vi "Image Processing with Vision Assistant (FPGA)test.vi"() -> ()   [LabVIEW 2016]
uses:
  <vilib>/visionFPGA/Controls/IMAQ FPGA Image Size.ctl
  <vilib>/rvi/Emulation/niFpgaSctlEmulationGetInTimedLoop.vi
  <vilib>/rvi/Emulation/niFpgaProcessEmulError.vi
  <vilib>/rvi/Emulation/niFpgaGetClockAttributes.vi
  <vilib>/rvi/Emulation/niFpgaEmulationReportErrorSimple.vi
  <vilib>/visionFPGA/Basics/FIFO to Pixel Bus/IMAQ FPGA FIFO to Pixel Bus RGB32x1.vi
  <vilib>/rvi/DataTransferAndStorage/Container/Common/niFpgaContainerGetUniqueNameForEmu.vi
  <vilib>/rvi/DataTransferAndStorage/Container/Common/niFpgaContainerSetEmuInfo.vi
  <vilib>/rvi/eio/common/nirviEmuReportErrorAndStop.vi
  <vilib>/rvi/interface/RandomDataEmulation/niFpgaRandomDataHandleErrors.vi
  <vilib>/rvi/Emulation/niFpgaCriticalErrorInLSC.vi
  <vilib>/rvi/LocalResourceManager/LocalResourceManager.xnode
  <vilib>/rvi/DataTransferAndStorage/Container/XNode/niFpgaContainer.xnode
  <vilib>/rvi/interface/RandomDataEmulation/nirviRandomDataFpgaReadWriteTemplate.vi
  <vilib>/visionFPGA/NI_VDM_FPGA_Basics.lvlib
panel:
  out "Output Valid":bool
  out "Ready For Output":bool=TRUE
  out "StartOfImage":bool=TRUE
  in  "Image Size":T1={"Width"=640, "Height"=480}
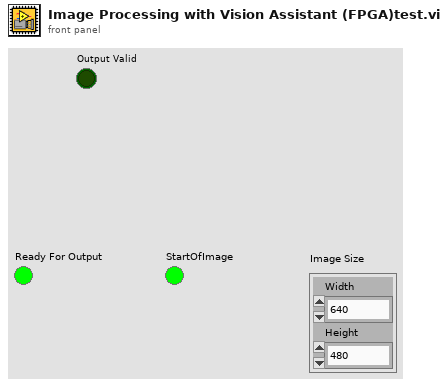
[diagram p1: front panel]
types:
  T1 = typedef "IMAQ FPGA Image Size.ctl" = cluster{"Width":u32, "Height":u32}
  T2 = typedef "IMAQ FPGA Pixel Bus RGB32x1.ctl" = cluster{"Pixel Data":cluster{"A":u8, "R/H":u8, "G/S":u8, "B/L":u8}, "DV":bool, "EOL":bool, "EOI":bool, "Data Type":enum16{"RGB32 x 1"}}
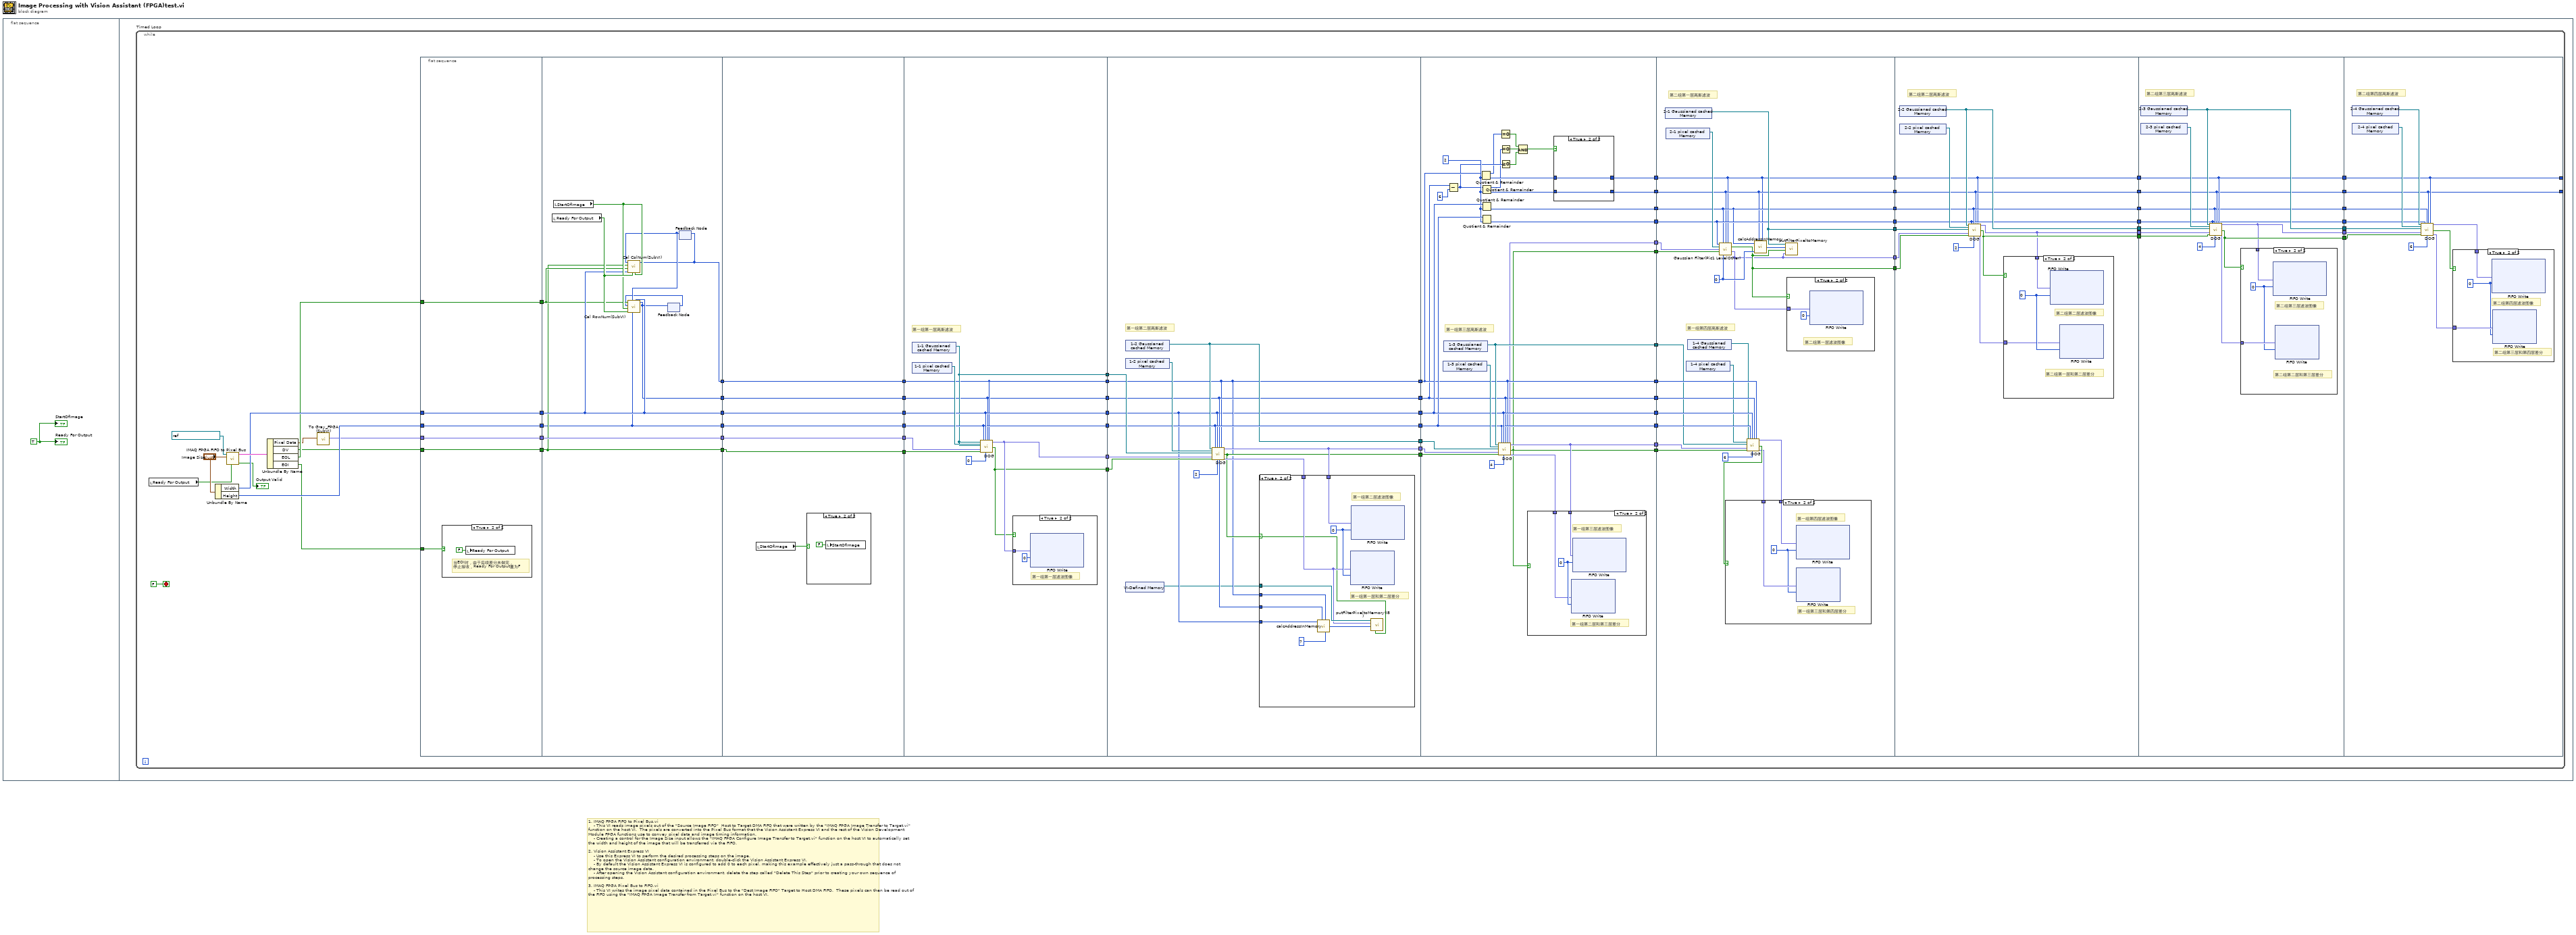
[diagram p0: block diagram]
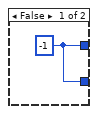
[diagram p6: hidden frame]
diagram:
  # "1. IMAQ FPGA FIFO to Pixel Bus.vi\n    - This VI reads image pixels out of the \"Source Image FIFO\"  Host to Target DMA FIFO that were written by the \"IMAQ FPGA Image Transfer to Target.vi\" function on the host VI.  The pixels are converted into the Pixel Bus format that the Vision Assistant Express VI and the rest of the Vision Development Module FPGA functions use to convey pixel data and image timing information.\n    - Creating a control for the Image Size input allows the \"IMAQ FPGA Configure Image Transfer to Target.vi\" function on the host VI to automatically set the width and height of the image that will be transferred via the FIFO.\n\n2. Vision Assistant Express VI\n    - Use this Express VI to perform the desired processing steps on the image.\n    - To open the Vision Assistant configuration environment, double-click the Vision Assistant Express VI.\n    - By default the Vision Assistant Express VI is configured to add 0 to each pixel, making this example effectively just a pass-through that does not change the source image data.\n    - After opening the Vision Assistant configuration environment, delete the step called \"Delete This Step\" prior to creating your own sequence of processing steps.\n\n3. IMAQ FPGA Pixel Bus to FIFO.vi\n    - This VI writes the image pixel data contained in the Pixel Bus to the \"Dest Image FIFO\" Target to Host DMA FIFO.  These pixels can then be read out of the FIFO using the \"IMAQ FPGA Image Transfer from Target.vi\" function on the host VI."
  n1 = flat-sequence {
    frame #0 {
      w1 = TRUE ("Ready For Output")
      "StartOfImage" <- w1
      "Ready For Output" <- w1
    }
    frame #1 {
      n2 = while "Timed Loop" {
        stop <- FALSE stop-if-true
        n3 = local read "Ready For Output"() -> (w12:bool)
        n4 = Unbundle By Name("Image Size") -> ("Width"=w68:u32, "Height"=w76:u32)
        n5 = call-poly <vilib>:"IMAQ FPGA FIFO to Pixel Bus.vi"("Ready For Output"=w12, "Image Size"="Image Size", "Source Image FIFO"=refnum<k21> "32it Source FIFO") -> ("Output Valid"=→"Output Valid":bool, "Pixel Bus Out"=w78:T2)  [unwired: 6 in, 1 out]
        n6 = Unbundle By Name(w78) -> ("Pixel Data"=w3:cluster{"A":u8, "R/H":u8, "G/S":u8, "B/L":u8}, "DV"=w2:bool, "EOL"=w13:bool, "EOI"=w75:bool)
        n7 = call "To Gray_FPGA (SubVI).vi"("Pixel Data"=w3) -> ("Data Out"=w4:fxp<+,8,8>)  [unwired: 10 in]
        n8 = flat-sequence {
          tunnel: w13 -> [w81]
          tunnel: w75 -> [w80]
          tunnel: w2 -> [w82]
          tunnel: w76 -> [w83]
          tunnel: w68 -> [w84]
          tunnel: w4 -> [w85]
          tunnel: [w85] -> w11
          tunnel: [w84] -> w10
          tunnel: [w83] -> w9
          tunnel: [w82] -> w8
          tunnel: [w81] -> w7
          tunnel: [w89] -> w19
          tunnel: [w87] -> w18
          tunnel: [w97] -> w17
          tunnel: [w94] -> w16
          tunnel: [w91] -> w15
          tunnel: [w92] -> w14
          tunnel: w11 -> [w97]
          tunnel: w10 -> [w94]
          tunnel: w9 -> [w91]
          tunnel: w8 -> [w92]
          tunnel: w7 -> [w93]
          tunnel: [w98] -> w74
          tunnel: [w104] -> w73
          tunnel: [w102] -> w72
          tunnel: [w103] -> w71
          tunnel: [w100] -> w70
          tunnel: [w99] -> w69
          tunnel: w19 -> [w99]
          tunnel: w18 -> [w100]
          tunnel: w17 -> [w104]
          tunnel: w16 -> [w103]
          tunnel: w15 -> [w102]
          tunnel: w14 -> [w98]
          tunnel: w74 -> [w115]
          tunnel: w73 -> [w116]
          tunnel: w72 -> [w111]
          tunnel: w71 -> [w112]
          tunnel: w70 -> [w107]
          tunnel: w69 -> [w106]
          tunnel: [w107] -> w67
          tunnel: [w106] -> w66
          tunnel: [w112] -> w65
          tunnel: [w111] -> w64
          tunnel: [w114] -> w63
          tunnel: [w108] -> w62
          tunnel: [w109] -> w59
          tunnel: w67 -> [w121]
          tunnel: w66 -> [w126]
          tunnel: w65 -> [w120]
          tunnel: w64 -> [w128]
          tunnel: w63 -> [w130]
          tunnel: w62 -> [w129]
          tunnel: [w123] -> w61
          tunnel: [w125] -> w60
          tunnel: w59 -> [w131]
          tunnel: [w121] -> w58
          tunnel: [w126] -> w57
          tunnel: [w120] -> w56
          tunnel: [w128] -> w55
          tunnel: [w127] -> w47
          tunnel: w61 -> [w171]
          tunnel: w60 -> [w170]
          tunnel: w58 -> [w159]
          tunnel: w57 -> [w158]
          tunnel: w56 -> [w164]
          tunnel: w55 -> [w162]
          tunnel: [w146] -> w54
          tunnel: [w144] -> w53
          tunnel: [w159] -> w52
          tunnel: [w158] -> w51
          tunnel: [w164] -> w50
          tunnel: [w162] -> w49
          tunnel: [w168] -> w48
          tunnel: w47 -> [w167]
          tunnel: [w163] -> w46
          tunnel: [w160] -> w45
          tunnel: [w152] -> w44
          tunnel: [w153] -> w43
          tunnel: [w146] -> w42
          tunnel: [w144] -> w41
          tunnel: w54 -> [w202]
          tunnel: w53 -> [w201]
          tunnel: w52 -> [w200]
          tunnel: w51 -> [w199]
          tunnel: w50 -> [w198]
          tunnel: w49 -> [w197]
          tunnel: w48 -> [w194]
          tunnel: w46 -> [w185]
          tunnel: w45 -> [w186]
          tunnel: w44 -> [w184]
          tunnel: w43 -> [w183]
          tunnel: w42 -> [w188]
          tunnel: w41 -> [w189]
          tunnel: [w191] -> w40
          tunnel: [w180] -> w39
          tunnel: [w181] -> w38
          tunnel: [w186] -> w37
          tunnel: [w185] -> w36
          tunnel: [w184] -> w35
          tunnel: [w183] -> w34
          tunnel: w40 -> [w218]
          tunnel: w39 -> [w217]
          tunnel: w38 -> [w216]
          tunnel: w37 -> [w213]
          tunnel: w36 -> [w214]
          tunnel: w35 -> [w212]
          tunnel: w34 -> [w211]
          tunnel: [w215] -> w33
          tunnel: [w211] -> w32
          tunnel: [w212] -> w31
          tunnel: [w214] -> w30
          tunnel: [w213] -> w29
          tunnel: [w208] -> w28
          tunnel: [w210] -> w27
          tunnel: w33 -> [w234]
          tunnel: w32 -> [w230]
          tunnel: w31 -> [w229]
          tunnel: w30 -> [w228]
          tunnel: w29 -> [w227]
          tunnel: w28 -> [w233]
          tunnel: w27 -> [w232]
          tunnel: [w225] -> w26
          tunnel: [w226] -> w25
          tunnel: [w231] -> w24
          tunnel: [w230] -> w23
          tunnel: [w229] -> w22
          tunnel: [w228] -> w21
          tunnel: [w227] -> w20
          tunnel: w26 -> [w249]
          tunnel: w25 -> [w248]
          tunnel: w24 -> [w247]
          tunnel: w23 -> [w244]
          tunnel: w22 -> [w243]
          tunnel: w21 -> [w246]
          tunnel: w20 -> [w245]
          tunnel: [w244] -> _
          tunnel: [w243] -> _
          frame #0 {
            n9 = case shown="True" w80 {
              frame False {
              }
              frame True {
                # "当EOI时，由于后续差分未做完，\n停止接收，Ready For Output置为F"
                n10 = local write "Ready For Output"(FALSE ("Ready For Output")) -> ()
              }
            }
          }
          frame #1 {
            n11 = local read "Ready For Output"() -> (w96:bool)
            n12 = local read "StartOfImage"() -> (w95:bool)
            n13 = feedback #1() -> (w88:u16)  [unwired: 1 in]
            n14 = feedback #2() -> (w90:u16)  [unwired: 1 in]
            n15 = call "Cal ColNum(SubVI).vi"("StartOfImage"=w95, "Ready For Input"=w96, "Width"=w94, "EOL"=w93, "DV"=w92, "curColNum"=w90) -> ("nextColNum"=w87:u16)  [unwired: 5 in]
            n16 = call "Cal RowNum(SubVI).vi"("Width"=w94, "Height"=w91, "curCol"=w90, "Ready For Input"=w96, "startOfImage"=w95, "curRow"=w88, "EOL"=w93) -> ("nextRow"=w89:u16)  [unwired: 4 in]
            n17 = feedback-in #1(w89) -> ()
            n18 = feedback-in #2(w87) -> ()
          }
          frame #2 {
            n19 = local read "StartOfImage"() -> (w101:bool)
            n20 = case shown="True" w101 {
              frame False {
              }
              frame True {
                n21 = local write "StartOfImage"(FALSE ("StartOfImage")) -> ()
              }
            }
          }
          frame #3 {
            # "第一组第一层高斯滤波"
            n22 = xnode "1-1 Gaussianed cached Memory"() -> ("Memory Out"=w109:refnum<k21>)
            n23 = xnode "1-1 pixel cached Memory"() -> ("Memory Out"=w113:refnum<k21>)
            n24 = call "DOG.vi"("Gaussianed cached Memory"=w109, "pixel cached Memory"=w113, "preGaussianed cached Memory"=w109, "Data in"=w116, "DV in"=w115, "Height"=w111, "Width"=w112, "DelayRowCount"=i16 0, "Rows"=w106, "Cols"=w107) -> ("GaussianFilterData out"=w114:fxp<+,12,12>, "DV out"=w108:bool)  [unwired: 6 in, 2 out]
            n25 = case shown="True" w108 {
              tunnel: w114 -> [_ w117]
              frame False {
              }
              frame True {
                # "第一组第一层滤波图像"
                n26 = xnode ("FIFO Write")("Element"=w117, "Timeout"=0) -> ()  [unwired: 1 in, 2 out]
              }
            }
          }
          frame #4 {
            # "第一组第二层高斯滤波"
            n27 = xnode "1-2 Gaussianed cached Memory"() -> ("Memory Out"=w127:refnum<k21>)
            n28 = xnode "1-2 pixel cached Memory"() -> ("Memory Out"=w132:refnum<k21>)
            n29 = xnode "VI-Defined Memory"() -> ("Memory Out"=w119:refnum<k21>)
            n30 = call "DOG.vi"("Gaussianed cached Memory"=w127, "pixel cached Memory"=w132, "preGaussianed cached Memory"=w131, "Data in"=w130, "DV in"=w129, "Height"=w128, "Width"=w120, "DelayRowCount"=i16 2, "Rows"=w126, "Cols"=w121) -> ("out Row"=w122:u16, "GaussianFilterData out"=w125:fxp<+,12,12>, "DV out"=w123:bool, "DOG Out"=w124:fxp<+/-,13,13>)  [unwired: 6 in]
            n31 = case shown="True" w123 {
              selector: w123 -> [_ w134]
              tunnel: w125 -> [_ w142]
              tunnel: w124 -> [_ w136]
              tunnel: w122 -> [_ w141]
              tunnel: w121 -> [_ w140]
              tunnel: w120 -> [_ w139]
              tunnel: w119 -> [_ w137]
              frame False {
              }
              frame True {
                w143 = 0 ("Timeout")
                # "第一组第一层和第二层差分"
                # "第一组第二层滤波图像"
                n32 = call "calcAddressInMemory.vi"("Width"=w139, "Rows"=w141, "Cols"=w140, "divider"=u8 7) -> ("addressInMemory"=w135:u16)  [unwired: 5 in]
                n33 = xnode ("FIFO Write")("Element"=w136, "Timeout"=w143) -> ()  [unwired: 1 in, 2 out]
                n34 = xnode ("FIFO Write")("Element"=w142, "Timeout"=w143) -> ()  [unwired: 1 in, 2 out]
                n35 = call "putFilterPixeltoMemory(I8).vi"("DV in"=w134, "addressInMemory"=w135, "Data In"=w136, "Memory in"=w137) -> ()  [unwired: 8 in]
              }
            }
          }
          frame #5 {
            w161 = u32 2 ("y")
            # "第一组第三层高斯滤波"
            n36 = xnode "1-3 pixel cached Memory"() -> ("Memory Out"=w169:refnum<k21>)
            n37 = xnode "1-3 Gaussianed cached Memory"() -> ("Memory Out"=w168:refnum<k21>)
            n38 = Subtract(x=w158, y=i16 6) -> (x-y=w149:u16)
            n39 = Quotient & Remainder(x=w159, y=w161) -> (x-y*floor(x/y)=w148:u32, floor(x/y)=w150:u32)
            n40 = Quotient & Remainder(x=w149, y=w161) -> (x-y*floor(x/y)=w147:u32, floor(x/y)=w151:u32)
            n41 = Quotient & Remainder(x=w164, y=w161) -> (floor(x/y)=w163:u32)  [unwired: 1 out]
            n42 = Quotient & Remainder(x=w162, y=w161) -> (floor(x/y)=w160:u32)  [unwired: 1 out]
            n43 = call "DOG.vi"("Gaussianed cached Memory"=w168, "pixel cached Memory"=w169, "preGaussianed cached Memory"=w167, "Data in"=w170, "DV in"=w171, "Height"=w162, "Width"=w164, "DelayRowCount"=i16 4, "Rows"=w158, "Cols"=w159) -> ("GaussianFilterData out"=w146:fxp<+,12,12>, "DV out"=w144:bool, "DOG Out"=w145:fxp<+/-,13,13>)  [unwired: 6 in, 1 out]
            n44 = Equal To 0?(x=w148) -> (x = 0?=w157:bool)
            n45 = Equal To 0?(x=w147) -> (x = 0?=w156:bool)
            n46 = Greater Or Equal To 0?(x=w149) -> (x >= 0?=w155:bool)
            n47 = Compound Arithmetic op=AND(w157, w156, w155) -> (w154:bool)
            n48 = case shown="True" w144 {
              tunnel: w146 -> [_ w176]
              tunnel: w145 -> [_ w175]
              frame False {
              }
              frame True {
                w177 = 0 ("Timeout")
                # "第一组第二层和第三层差分"
                # "第一组第三层滤波图像"
                n49 = xnode ("FIFO Write")("Element"=w175, "Timeout"=w177) -> ()  [unwired: 1 in, 2 out]
                n50 = xnode ("FIFO Write")("Element"=w176, "Timeout"=w177) -> ()  [unwired: 1 in, 2 out]
              }
            }
            n51 = case shown="True" w154 {
              tunnel: [w172 w174] -> w153
              tunnel: w150 -> [_ w174]
              tunnel: [w172 w173] -> w152
              tunnel: w151 -> [_ w173]
              frame False {
                w172 = i16 -1 ("t")
              }
              frame True {
              }
            }
          }
          frame #6 {
            w182 = i16 0 ("delayRowCount")
            # "第二组第一层高斯滤波"
            # "第一组第四层高斯滤波"
            n52 = xnode "2-1 Gaussianed cached Memory"() -> ("Memory Out"=w191:refnum<k21>)
            n53 = xnode "2-1 pixel cached Memory"() -> ("Memory Out"=w187:refnum<k21>)
            n54 = xnode "1-4 pixel cached Memory"() -> ("Memory Out"=w195:refnum<k21>)
            n55 = xnode "1-4 Gaussianed cached Memory"() -> ("Memory Out"=w196:refnum<k21>)
            n56 = call "Gaussian Filter(Pic1 LevelOther).vi"("Height"=w186, "Width"=w185, "Rows"=w184, "Cols"=w183, "Memory in"=w187, "Data in"=w188, "DV in"=w189, "DelayRowCount"=w182) -> ("DV out"=w181:bool, "Data Out"=w180:fxp<+,8,8>)  [unwired: 5 in, 1 out]
            n57 = call "DOG.vi"("Gaussianed cached Memory"=w196, "pixel cached Memory"=w195, "preGaussianed cached Memory"=w194, "Data in"=w202, "DV in"=w201, "Height"=w197, "Width"=w198, "DelayRowCount"=i16 6, "Rows"=w199, "Cols"=w200) -> ("GaussianFilterData out"=w190:fxp<+,12,12>, "DV out"=w179:bool, "DOG Out"=w178:fxp<+/-,13,13>)  [unwired: 6 in, 1 out]
            n58 = case shown="True" w179 {
              tunnel: w190 -> [_ w207]
              tunnel: w178 -> [_ w206]
              frame False {
              }
              frame True {
                w205 = 0 ("Timeout")
                # "第一组第三层和第四层差分"
                # "第一组第四层滤波图像"
                n59 = xnode ("FIFO Write")("Element"=w207, "Timeout"=w205) -> ()  [unwired: 1 in, 2 out]
                n60 = xnode ("FIFO Write")("Element"=w206, "Timeout"=w205) -> ()  [unwired: 1 in, 2 out]
              }
            }
            n61 = call "calcAddressInMemory.vi"("Width"=w185, "Rows"=w184, "delayRowCount"=w182, "Cols"=w183) -> ("addressInMemory"=w192:u16)  [unwired: 5 in]
            n62 = call "putFilterPixeltoMemory.vi"("Data In"=w180, "DV in"=w181, "addressInMemory"=w192, "Memory in"=w191) -> ()
            n63 = case shown="True" w181 {
              tunnel: w180 -> [_ w203]
              frame False {
              }
              frame True {
                # "第二组第一层滤波图像"
                n64 = xnode ("FIFO Write")("Element"=w203, "Timeout"=0) -> ()  [unwired: 1 in, 2 out]
              }
            }
          }
          frame #7 {
            # "第二组第二层高斯滤波"
            n65 = xnode "2-2 Gaussianed cached Memory"() -> ("Memory Out"=w215:refnum<k21>)
            n66 = xnode "2-2 pixel cached Memory"() -> ("Memory Out"=w219:refnum<k21>)
            n67 = call "DOG.vi"("Gaussianed cached Memory"=w215, "pixel cached Memory"=w219, "preGaussianed cached Memory"=w218, "Data in"=w217, "DV in"=w216, "Height"=w213, "Width"=w214, "DelayRowCount"=i16 2, "Rows"=w212, "Cols"=w211) -> ("GaussianFilterData out"=w208:fxp<+,12,12>, "DV out"=w210:bool, "DOG Out"=w209:fxp<+/-,13,13>)  [unwired: 6 in, 1 out]
            n68 = case shown="True" w210 {
              tunnel: w209 -> [_ w222]
              tunnel: w208 -> [_ w221]
              frame False {
              }
              frame True {
                w223 = 0 ("Timeout")
                # "第二组第一层和第二层差分"
                # "第二组第二层滤波图像"
                n69 = xnode ("FIFO Write")("Element"=w221, "Timeout"=w223) -> ()  [unwired: 1 in, 2 out]
                n70 = xnode ("FIFO Write")("Element"=w222, "Timeout"=w223) -> ()  [unwired: 1 in, 2 out]
              }
            }
          }
          frame #8 {
            # "第二组第三层高斯滤波"
            n71 = xnode "2-3 Gaussianed cached Memory"() -> ("Memory Out"=w231:refnum<k21>)
            n72 = xnode "2-3 pixel cached Memory"() -> ("Memory Out"=w235:refnum<k21>)
            n73 = call "DOG.vi"("Gaussianed cached Memory"=w231, "pixel cached Memory"=w235, "preGaussianed cached Memory"=w234, "Data in"=w233, "DV in"=w232, "Height"=w227, "Width"=w228, "DelayRowCount"=i16 4, "Rows"=w229, "Cols"=w230) -> ("GaussianFilterData out"=w225:fxp<+,12,12>, "DV out"=w226:bool, "DOG Out"=w224:fxp<+/-,13,13>)  [unwired: 6 in, 1 out]
            n74 = case shown="True" w226 {
              tunnel: w225 -> [_ w239]
              tunnel: w224 -> [_ w238]
              frame False {
              }
              frame True {
                w237 = 0 ("Timeout")
                # "第二组第二层和第三层差分"
                # "第二组第三层滤波图像"
                n75 = xnode ("FIFO Write")("Element"=w239, "Timeout"=w237) -> ()  [unwired: 1 in, 2 out]
                n76 = xnode ("FIFO Write")("Element"=w238, "Timeout"=w237) -> ()  [unwired: 1 in, 2 out]
              }
            }
          }
          frame #9 {
            # "第二组第四层高斯滤波"
            n77 = xnode "2-4 Gaussianed cached Memory"() -> ("Memory Out"=w250:refnum<k21>)
            n78 = xnode "2-4 pixel cached Memory"() -> ("Memory Out"=w251:refnum<k21>)
            n79 = call "DOG.vi"("Gaussianed cached Memory"=w250, "pixel cached Memory"=w251, "preGaussianed cached Memory"=w247, "Data in"=w249, "DV in"=w248, "Height"=w245, "Width"=w246, "DelayRowCount"=i16 6, "Rows"=w243, "Cols"=w244) -> ("GaussianFilterData out"=w241:fxp<+,12,12>, "DV out"=w242:bool, "DOG Out"=w240:fxp<+/-,13,13>)  [unwired: 6 in, 1 out]
            n80 = case shown="True" w242 {
              tunnel: w241 -> [_ w255]
              tunnel: w240 -> [_ w254]
              frame False {
              }
              frame True {
                w253 = 0 ("Timeout")
                # "第二组第三层和第四层差分"
                # "第二组第四层滤波图像"
                n81 = xnode ("FIFO Write")("Element"=w255, "Timeout"=w253) -> ()  [unwired: 1 in, 2 out]
                n82 = xnode ("FIFO Write")("Element"=w254, "Timeout"=w253) -> ()  [unwired: 1 in, 2 out]
              }
            }
          }
        }
      }
    }
  }
